vi "Create Log File.vi"(8 "error in (no error)":errorcluster, 11 "Acceleration Exceeded Log Folder":path=path "c:/logfiles") -> (0 "error out":errorcluster, 3 "Log File out":refnum<k34>)   [LabVIEW 2017, in "Logging.lvlib"]
uses:
  Logging.lvlib
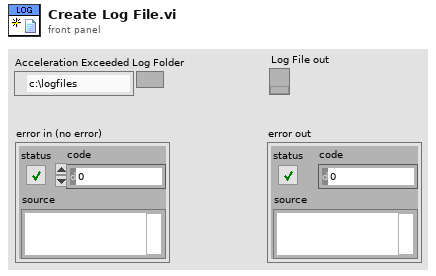
[diagram p1: front panel]
types:
  T1 = enum16{"open", "open or create", "create or replace", "create", "open (read-only)"}
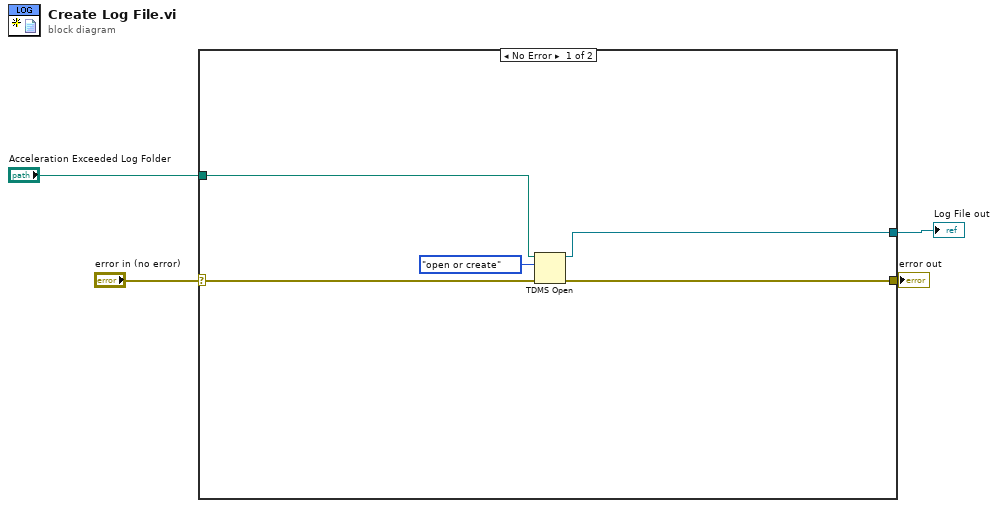
[diagram p0: block diagram]
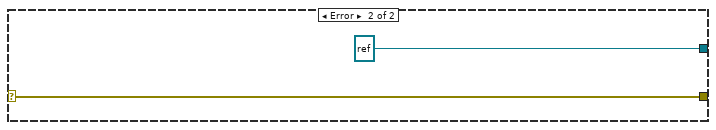
[diagram p2: hidden frame]
diagram:
  n1 = case shown="No Error" "error in (no error)" {
    selector: "error in (no error)" -> [w7 w10]
    tunnel: [w9 refnum<k34> refnum ("tdms file out")] -> w4
    tunnel: "Acceleration Exceeded Log Folder" -> [w6 _]
    tunnel: [w8 w10] -> w1
    frame No Error {
      n2 = TDMS Open(8:w7, 10:T1."open or create" ("operation (0:open)"), 11:w6) -> (0:w8:errorcluster, 3:w9:refnum<k34>)  [unwired: 4 in]
    }
    frame Error {
    }
  }
  "Log File out" <- w4
  "error out" <- w1
